vi "Read Request Headers.vi"(8 "error in (no error)":errorcluster, 11 "REST Interface in":refnum<class "REST Interface.lvclass">) -> (0 "error out":errorcluster, 2 "Request Headers":T1[](array[typedef]), 3 "REST Interface out":refnum<class "REST Interface.lvclass">)   [LabVIEW 2018, in "REST Interface.lvlib" / "REST Interface.lvclass"]
uses:
  REST Interface.lvclass
  <vilib>/addons/_JKI.lib/REST Client/classes/REST Client/HTTP Header.ctl
  REST Interface.lvclass/REST Interface.ctl
  <vilib>/addons/_JKI.lib/REST Client/classes/REST Client/REST Client.lvclass
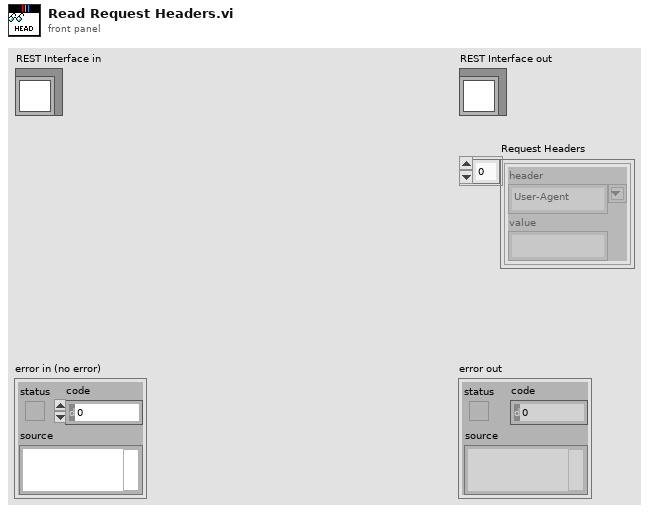
[diagram p1: front panel]
types:
  T1 = typedef "REST Client.lvlib/REST Client.lvclass/HTTP Header.ctl" = cluster{"header":string, "value":string}
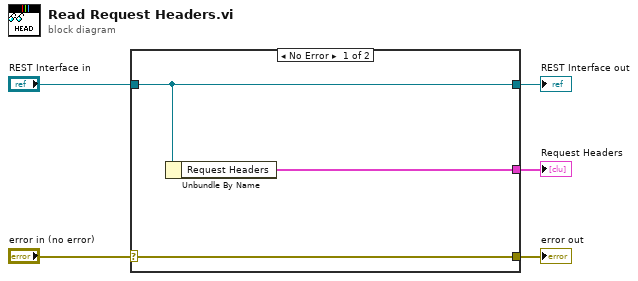
[diagram p0: block diagram]
diagram:
  n1 = case shown="No Error" "error in (no error)" {
    selector: "error in (no error)" -> [w8 w9]
    tunnel: [w8 w9] -> w4
    tunnel: [w7 w10] -> w2
    tunnel: "REST Interface in" -> [w7 w10]
    tunnel: [w6 _] -> w1
    frame No Error {
      n2 = Unbundle By Name(w7) -> ("Request Headers"=w6:T1[])
    }
    frame Error {
    }
  }
  "error out" <- w4
  "REST Interface out" <- w2
  "Request Headers" <- w1
